vi "Oxford.vi"() -> ()   [LabVIEW 2019]
panel:
  out "?":string[](array[string])
  in  "?":u16[](array[ring])=[6, 0, 1] items=["Demand current (Output current) (A)", "Measured power supply voltage (V)", "Measured magnet current (A)", "Demand current (Duplicate) (A)", "Set point (A)", "Sweep rate (A/min)", "Demand Field (Output Field ) (T)", "Set point (T)", "Sweep rate (T/min)", "Lead resistance (milli ohms)", "Channel 1 freq/4", "Channel 2 freq/4", "Channel 3 freq/4", "PSU zero correction (Hex)", "Software voltage limit (V)", "Persistent magnet current (A)", "Trip current (A)", "Persistent magnet Field (T)", "Trip field (T)", "Demand current as a Hex number", "Safe current limit, Most negative (A)", "Safe current limit, Most positive (A)"]
  in  "?":bool=TRUE
  out "Error: Illegal command\nor\nIllegal sequence of commands":bool
  out "Current persistent field (T):":string
  out "Output Voltage":dbl(knob) scale=-20.0..20.0 scale format="%.1f"
  in  "?":u32(slide) scale=0.0..3.0
  out "Heater output":bool
  out "Output Current":dbl(knob) scale=-10.0..10.0 scale format="%.1f"
  in  "Ramp rate (A/min):":dbl=2.0 min=0.0 max=500.0 step=0.2 format="%.2f"
  in  "Set Point (T):":dbl min=0.0 max=17.5 step=0.001 format="%.3f"
  in  "?":u32(slide)=3 scale=0.0..3.0
  in  "?":u32(slide)=3 scale=0.0..3.0
  out "Rate limiting":bool
  out "Magnet Over Heated":bool
  out "Quenched":bool
  out "Magnet Warming up":bool
  out "Power supply status:":string
  out "Software Version":string
  in  "?":u32(slide) scale=0.0..2.0
  # "Diagnostic tools & Indicators"
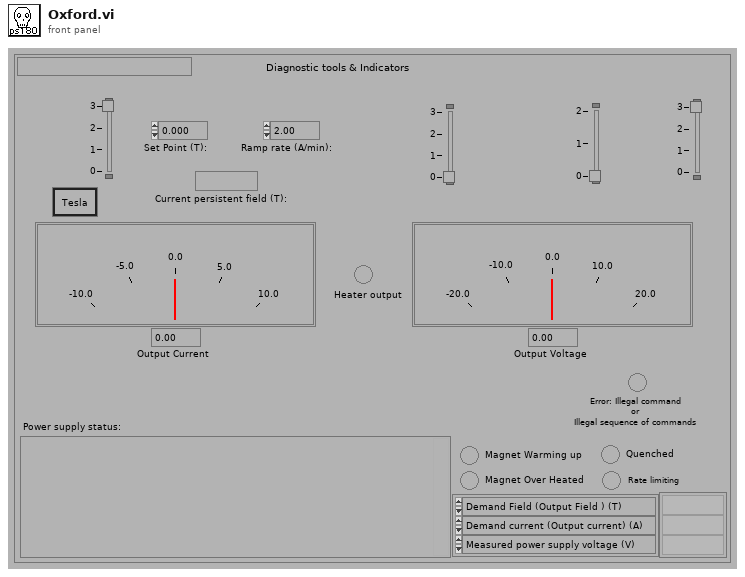
[diagram p1: front panel]
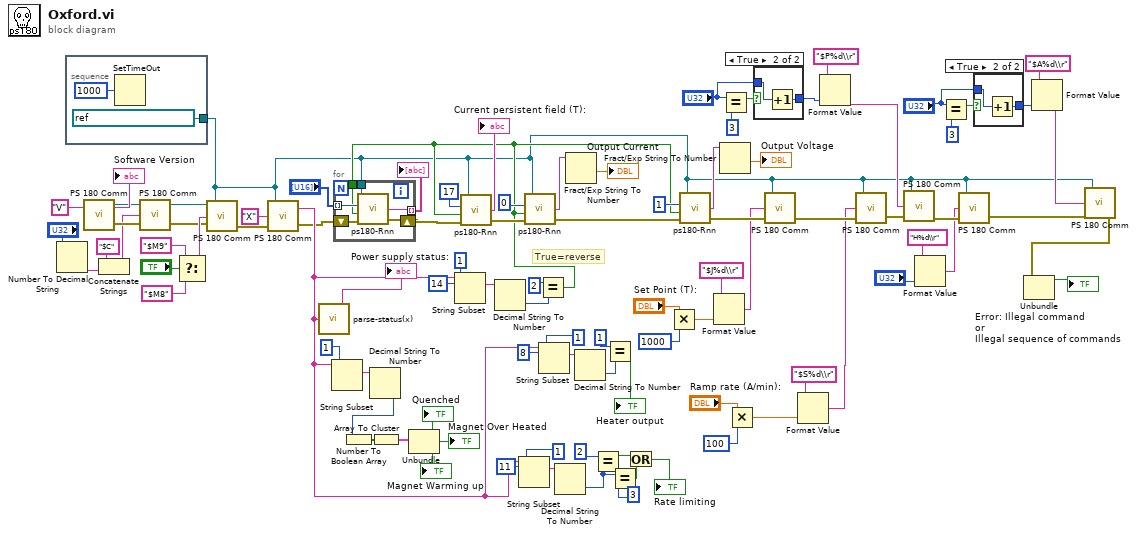
[diagram p0: block diagram]
diagram:
  w72 = 1
  # "True=reverse"
  n1 = Number To Decimal String(number="?") -> (decimal integer string=w87:string)  [unwired: 1 in]
  n2 = stacked-sequence {
    tunnel: [refnum<visa-resource-name> "GPIB0::24::INSTR" ("VISA session")] -> w1
    frame #0 {
      n3 = SetTimeOut(1:1000) -> ()  [unwired: 1 out]
    }
  }
  n4 = call "PS 180 Comm.vi"(3:"V", "VISA session"=w1) -> ("error out"=w90:errorcluster, 1:→"Software Version":string)  [unwired: 1 in]
  n5 = Concatenate Strings("$C", w87) -> (w86:string)
  n6 = call "PS 180 Comm.vi"("error in (no error)"=w90, 3:w86, "VISA session"=w1) -> ("error out"=w81:errorcluster)  [unwired: 1 out]
  n7 = Select(t="$M9", s="?", f="$M8") -> (s? t:f=w82:string)
  n8 = call "PS 180 Comm.vi"("error in (no error)"=w81, 3:w82, "VISA session"=w1) -> ("error out"=w79:errorcluster)  [unwired: 1 out]
  n9 = call "PS 180 Comm.vi"("error in (no error)"=w79, 3:"X", "VISA session"=w1) -> ("error out"=w54:errorcluster, 1:w55:string)
  n10 = call "parse-status(x).vi"("Writein the response of the ps180 to the Status command (X):"=w55) -> ("Status"=→"Power supply status:":string)
  n11 = String Subset(string=w55, offset (0)=w72, length (rest)=w72) -> (substring=w62:string)
  n12 = Decimal String To Number(string=w62) -> (number=w15:i32)  [unwired: 2 in, 1 out]
  n13 = Number To Boolean Array(number=w15) -> (Boolean array=w20:bool[])
  n14 = Array To Cluster(array=w20) -> (cluster=w19:cluster{"[0]":bool, "[1]":bool, "[2]":bool})
  n15 = Unbundle(w19) -> ("[0]"=→"Quenched":bool, "[1]"=→"Magnet Over Heated":bool, "[2]"=→"Magnet Warming up":bool)
  n16 = String Subset(string=w55, offset (0)=14, length (rest)=1) -> (substring=w58:string)
  n17 = Decimal String To Number(string=w58) -> (number=w61:i32)  [unwired: 2 in, 1 out]
  n18 = String Subset(string=w55, offset (0)=11, length (rest)=1) -> (substring=w70:string)
  n19 = Equal?(x=2, y=w61) -> (x = y?=w14:bool)
  n20 = for {
    shift-right: [w99] -> w51
    shift-left: w54 -> [w100]
    tunnel: "?" -> [w98] mode=indexing
    tunnel: [w97] -> w52 mode=indexing
    tunnel: w1 -> [w96]
    tunnel: w14 -> [w95]
    n21 = call "ps180-Rnn.vi"("error in (no error)"=w100, "Polarity"=w95, "Read parameter"=w98, "VISA session"=w96) -> ("error out"=w99:errorcluster, "Output string"=w97:string)  [unwired: 1 in]
  }
  "?" <- w52
  n22 = call "ps180-Rnn.vi"("error in (no error)"=w51, "Polarity"=w14, "Read parameter"=u16 17, "VISA session"=w1) -> ("error out"=w47:errorcluster, "Output string"=→"Current persistent field (T):":string)  [unwired: 1 in]
  n23 = call "ps180-Rnn.vi"("error in (no error)"=w47, "Polarity"=w14, "Read parameter"=u16 0, "VISA session"=w1) -> ("error out"=w44:errorcluster, "Output string"=w45:string)  [unwired: 1 in]
  n24 = String Subset(string=w55, offset (0)=8, length (rest)=1) -> (substring=w66:string)
  n25 = Decimal String To Number(string=w70) -> (number=w73:i32)  [unwired: 2 in, 1 out]
  n26 = Fract/Exp String To Number(string=w45) -> (number=→"Output Current":dbl)  [unwired: 3 in, 1 out]
  n27 = Decimal String To Number(string=w66) -> (number=w63:i32)  [unwired: 2 in, 1 out]
  n28 = Equal?(x=2, y=w73) -> (x = y?=w75:bool)
  n29 = Equal?(x=1, y=w63) -> (x = y?=→"Heater output":bool)
  n30 = Equal?(x=w73, y=3) -> (x = y?=w76:bool)
  n31 = Or(x=w75, y=w76) -> (x .or. y?=→"Rate limiting":bool)
  n32 = Multiply(x="Set Point (T):", y=1000) -> (x*y=w3:dbl)
  n33 = call "ps180-Rnn.vi"("error in (no error)"=w44, "Polarity"=w14, "Read parameter"=u16 1, "VISA session"=w1) -> ("error out"=w38:errorcluster, "Output string"=w42:string)  [unwired: 1 in]
  n34 = Format Value(format string="$J%d\\r", value (0)=w3) -> (output string=w2:string)  [unwired: 1 in]
  n35 = Fract/Exp String To Number(string=w42) -> (number=→"Output Voltage":dbl)  [unwired: 3 in, 1 out]
  n36 = Equal?(x="?", y=u32 3) -> (x = y?=w32:bool)
  n37 = Multiply(x="Ramp rate (A/min):", y=100) -> (x*y=w6:dbl)
  n38 = case shown="True" w32 {
    tunnel: [w101 w103] -> w13
    tunnel: "?" -> [w101 w102]
    frame False {
    }
    frame True {
      n39 = Increment(x=w102) -> (x+1=w103:u32)
    }
  }
  n40 = call "PS 180 Comm.vi"("error in (no error)"=w38, 3:w2, "VISA session"=w1) -> ("error out"=w35:errorcluster)  [unwired: 1 out]
  n41 = Format Value(format string="$S%d\\r", value (0)=w6) -> (output string=w5:string)  [unwired: 1 in]
  n42 = Format Value(format string="$P%d\\r", value (0)=w13) -> (output string=w12:string)  [unwired: 1 in]
  n43 = call "PS 180 Comm.vi"("error in (no error)"=w35, 3:w5, "VISA session"=w1) -> ("error out"=w31:errorcluster)  [unwired: 1 out]
  n44 = call "PS 180 Comm.vi"("error in (no error)"=w31, 3:w12, "VISA session"=w1) -> ("error out"=w30:errorcluster)  [unwired: 1 out]
  n45 = Format Value(format string="H%d\\r", value (0)="?") -> (output string=w9:string)  [unwired: 1 in]
  n46 = Equal?(x="?", y=u32 3) -> (x = y?=w29:bool)
  n47 = call "PS 180 Comm.vi"("error in (no error)"=w30, 3:w9, "VISA session"=w1) -> ("error out"=w23:errorcluster)  [unwired: 1 out]
  n48 = case shown="True" w29 {
    tunnel: [w104 w106] -> w26
    tunnel: "?" -> [w104 w105]
    frame False {
    }
    frame True {
      n49 = Increment(x=w105) -> (x+1=w106:u32)
    }
  }
  n50 = Format Value(format string="$A%d\\r", value (0)=w26) -> (output string=w24:string)  [unwired: 1 in]
  n51 = call "PS 180 Comm.vi"("error in (no error)"=w23, 3:w24, "VISA session"=w1) -> ("error out"=w21:errorcluster)  [unwired: 1 out]
  n52 = Unbundle(w21) -> ("status"=→"Error: Illegal command\nor\nIllegal sequence of commands":bool)  [unwired: 2 out]
